vi "布尔数据处理.vi"(9 "布尔输入":bool, 10 "行数":string, 11 "表格":string[][](table)) -> (3 "要发送的数据":cluster{"地址":u16, "数据":i32, "行数":i32, "ID":i32})   [LabVIEW 2021]
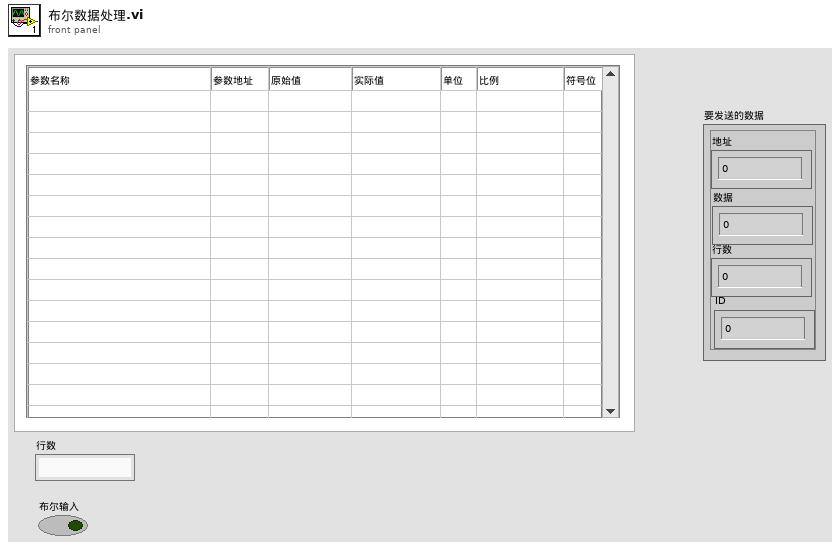
[diagram p1: front panel]
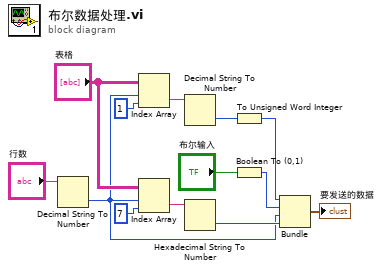
[diagram p0: block diagram]
diagram:
  n1 = Decimal String To Number(string="行数") -> (number=w2:i32)  [unwired: 2 in, 1 out]
  n2 = Index Array(array="表格", index (row)=w2, index (col)=1 ("禁用的索引 (列)")) -> (element=w11:string)
  n3 = Index Array(array="表格", index (row)=w2, index (col)=7 ("禁用的索引 (列)")) -> (element=w7:string)
  n4 = Decimal String To Number(string=w11) -> (number=w9:i32)  [unwired: 2 in, 1 out]
  n5 = Hexadecimal String To Number(string=w7) -> (number=w5:u32)  [unwired: 2 in, 1 out]
  n6 = To Unsigned Word Integer(number=w9) -> (unsigned 16bit integer=w13:u16)
  n7 = Boolean To (0,1)(Boolean="布尔输入") -> (0, 1=w12:i16)
  n8 = Bundle(w13, w12, w2, w5) -> (→"要发送的数据":cluster{u16, i16, i32, u32})  [unwired: 1 in]
